vi "read barometer.vi"(8 "error in (no error)":errorcluster) -> (0 "error out":errorcluster, 3 "function return":i32)   [LabVIEW 2014, in "libroboticscape.lvlib"]
doc: "int read_barometer();"
uses:
  libroboticscape.lvlib
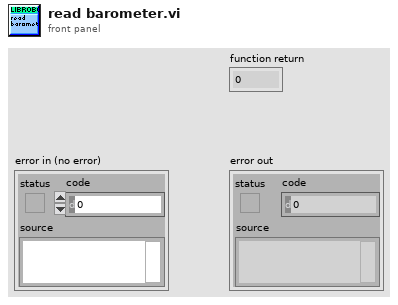
[diagram p1: front panel]
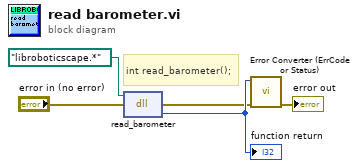
[diagram p0: block diagram]
diagram:
  # "int read_barometer();"
  n1 = dll-call lib="C:/Users/ktalke/Documents/Robotics-Cape-Master-Jessie/Libroboticscape-Master-Jessie/libroboticscape.so" fn="read_barometer"(path in=path "libroboticscape.*", error in="error in (no error)") -> (error out=w3:errorcluster, "return type"=w5:i32)  [unwired: 1 in, 1 out]
  "function return" <- w5
  n2 = call "Error Converter (ErrCode or Status).vi"("error in (no error)"=w3, "error code"=w5) -> ("error out"=→"error out":errorcluster)  [unwired: 9 in]
